vi "AnalogAcquiringVI.vi"(4 "Stage events":refnum<queue>, 6 "Image events":refnum<queue>, 7 "Microscope events":refnum<queue>, 8 "error in (no error)":errorcluster, 9 "raw data":refnum<queue>, 10 "X Data":refnum<queue>, 11 "Microscope in":refnum<class "Microscope.lvclass">) -> (0 "error out":errorcluster, 3 "Microscope out":refnum<class "Microscope.lvclass">)   [LabVIEW 2012, in "Microscope.lvclass"]
uses:
  classes/Microscope.lvclass
  typedefs/ImageEvent.ctl
  typedefs/StageEvent.ctl
  typedefs/MicroscopeEvent.ctl
  classes/Microscope.lvclass/Microscope.ctl
  variables/GlobalUI.vi
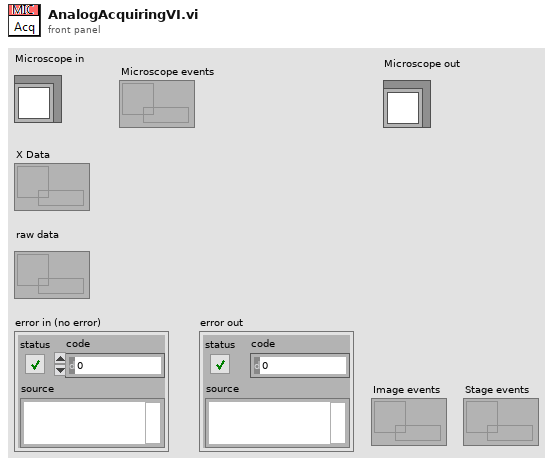
[diagram p1: front panel]
types:
  T1 = typedef "ImageEvent.ctl" = enum16{"i.Wait", "i.Acquire", "i.InitImageData", "i.ReinitImageData", "i.ReinitImageParams", "i.PreAcquire", "i.PostAcquire", "i.ClearData"}
  T2 = typedef "DetectorType.ctl" = enum16{"PMT", "SpectraWiz"}
  T3 = typedef "MicroscopeEvent.ctl" = enum16{"M.Wait", "M.RunRotation", "M.Flush", "M.Init", "M.InitStage", "M.InitImageData", "M.ReinitImageData", "M.ReinitImageParams", "M.GetSetParams", "M.InitFastHardware", "M.Pre-Acquire", "M.Acquire", "M.PostAcquire", "M.StopAcquire", "M.SetAcqStatusTrue", "M.SetAcqStatusFalse", "M.ClearImageData", "M.MoveStageDiscrete", "M.MoveStageToTarget1", "M.MoveStageToTarget2", "M.MoveStageToTarget3", "M.OpenShutters", "M.CloseShutters", "M.StartAcquireSequence", "M.ChangeParameters", "M.OpenStokes", "M.OpenPump", "M.RunSW"}
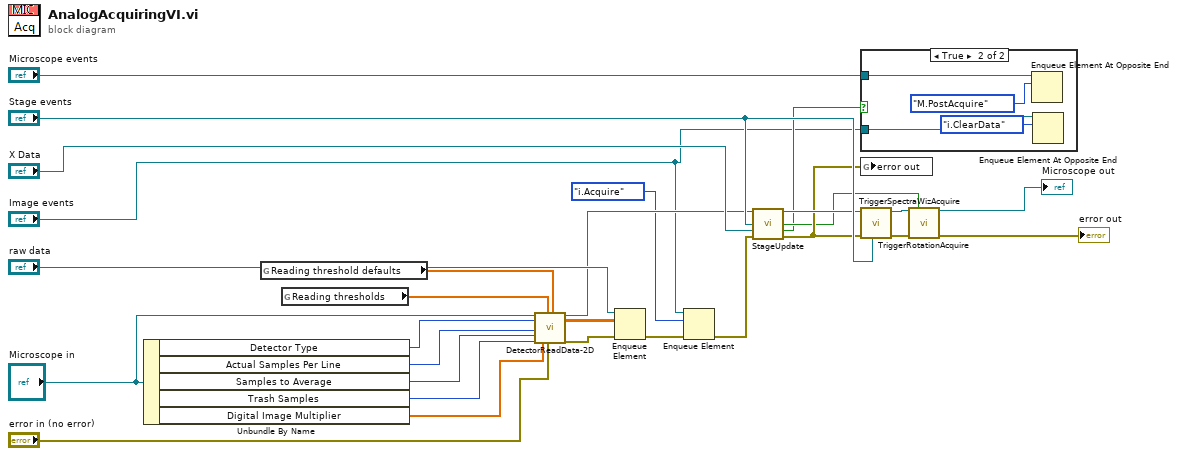
[diagram p0: block diagram]
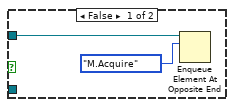
[diagram p2: hidden frame]
diagram:
  n1 = Unbundle By Name("Microscope in") -> ("Detector Type"=w25:T2, "Actual Samples Per Line"=w26:i32, "Samples to Average"=w24:i32, "Trash Samples"=w23:i32, "Digital Image Multiplier"=w4:dbl[])
  n2 = global read "GlobalUI.vi" "Reading threshold defaults"() -> (w2:dbl[])
  n3 = global read "GlobalUI.vi" "Reading thresholds"() -> (w3:dbl[])
  n4 = call "DetectorReadData-2D.vi"("Microscope in"="Microscope in", "Detector Type"=w25, "Actual Samples Per Line"=w26, "Computed Parameter.Samples to Average"=w24, "Computed Parameter.Trash Samples"=w23, "Digital Image Multiplier"=w4, "Threshold"=w3, "error in (no error)"="error in (no error)", "Threshold defaults"=w2) -> ("Microscope out"=w18:refnum<class "Microscope.lvclass">, "Data"=w11:dbl[][], "error out"=w12:errorcluster)  [unwired: 8 in]
  n5 = Enqueue Element(queue="raw data", element=w11, error in (no error)=w12) -> (error out=w13:errorcluster)  [unwired: 1 in, 2 out]
  n6 = Enqueue Element(queue="Image events", element=ImageEvent."i.Acquire", error in (no error)=w13) -> (error out=w8:errorcluster)  [unwired: 1 in, 2 out]
  n7 = call "StageUpdate.vi"("Microscope in"=w18, "Stage events"="Stage events", "X Data"="X Data", "error in (no error)"=w8) -> ("Microscope out"=w17:refnum<class "Microscope.lvclass">, "Image full"=w15:bool, "stop loop"=w7:bool, "error out"=w16:errorcluster)  [unwired: 8 in]
  n8 = case shown="True" w7 {
    tunnel: "Microscope events" -> [w30 w34]
    tunnel: "Image events" -> [_ w32]
    frame False {
      n9 = Enqueue Element At Opposite End(queue=w30, element=MicroscopeEvent."M.Acquire") -> ()  [unwired: 2 in, 3 out]
    }
    frame True {
      n10 = Enqueue Element At Opposite End(queue=w34, element=MicroscopeEvent."M.PostAcquire") -> ()  [unwired: 2 in, 3 out]
      n11 = Enqueue Element At Opposite End(queue=w32, element=ImageEvent."i.ClearData") -> ()  [unwired: 2 in, 3 out]
    }
  }
  n12 = global write "GlobalUI.vi" "error out"(w16) -> ()
  n13 = call "TriggerSpectraWizAcquire.vi"("Stage events"="Stage events", "error in (no error)"=w16, "Microscope in"=w17) -> ("error out"=w9:errorcluster, "Microscope out"=w10:refnum<class "Microscope.lvclass">)  [unwired: 7 in]
  n14 = call "TriggerRotationAcquire.vi"("Microscope in"=w10, "Trigger"=w15, "error in (no error)"=w9) -> ("Microscope out"=→"Microscope out":refnum<class "Microscope.lvclass">, "error out"=→"error out":errorcluster)  [unwired: 11 in]
